vi "flipping array.vi"() -> ()   [LabVIEW 2018]
panel:
  out "Array":dbl[][][](array[numeric])
  in  "Array - Numeric":dbl[](array[numeric])
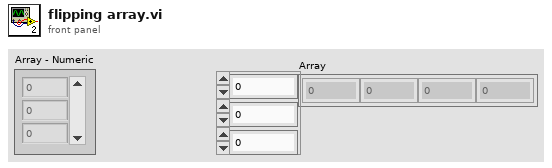
[diagram p1: front panel]
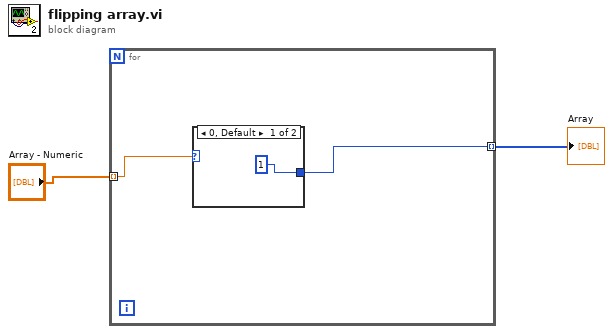
[diagram p0: block diagram]
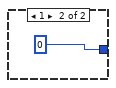
[diagram p2: hidden frame]
diagram:
  n1 = for {
    tunnel: "Array - Numeric" -> [w4] mode=indexing
    tunnel: [w3] -> w1 mode=indexing
    n2 = case shown="0, Default" w4 {
      tunnel: [1 0] -> w3
      frame 0, Default {
      }
      frame 1 {
      }
    }
  }
  "Array" <- w1
